vi "Acquire_PID_Tests.vi"() -> ()   [LabVIEW 2016]
panel:
  in  "Wait For Microscope?":bool
  in  "stop2":bool
  in  "Flow Path":path=path "E:/maggot images/Jacob/20171101/Flow_tests_run101.txt"
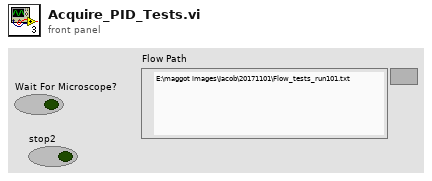
[diagram p1: front panel]
types:
  T1 = cluster{"relative seconds":dbl, "Pressures":dbl[], "F1 PID gains":dbl[], "FTot PID gains":dbl[], "PID On?":i16, "flow setpoints":dbl[]}
  T2 = cluster{"Time":dbl, "All Flow-Rates":dbl[], "Flow 2 Filter Time":dbl, "Flow 1 Filter Time":dbl}
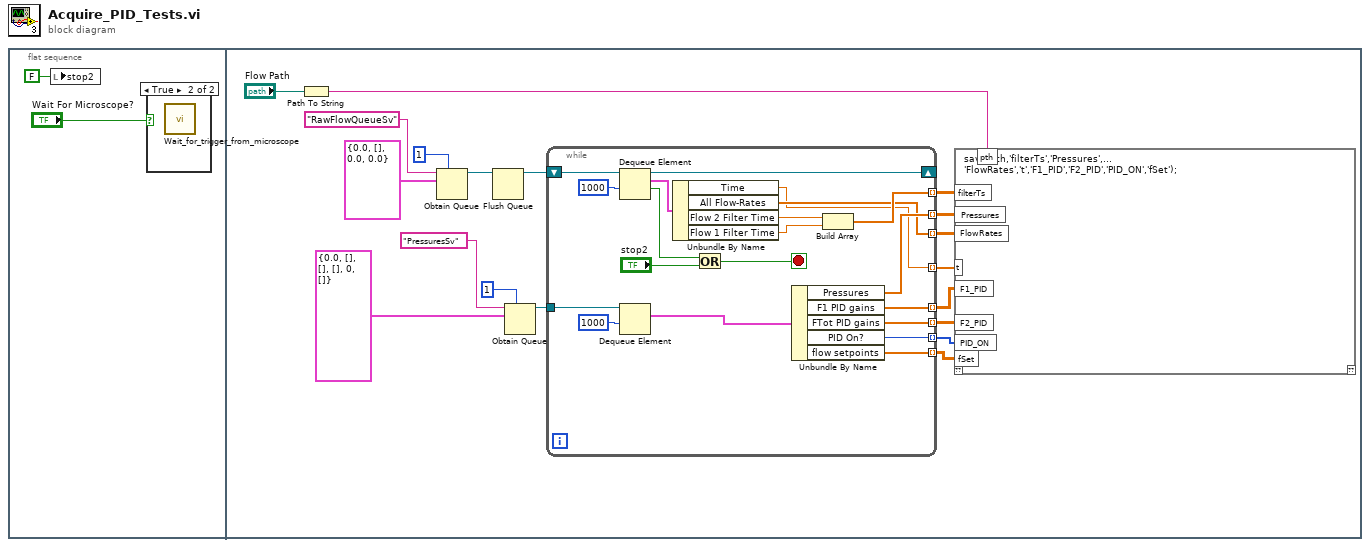
[diagram p0: block diagram]
diagram:
  n1 = flat-sequence {
    frame #0 {
      n2 = local write "stop2"(FALSE ("stop2")) -> ()
      n3 = case shown="True" "Wait For Microscope?" {
        frame False {
        }
        frame True {
          n4 = call "Wait_for_trigger_from_microscope.vi"() -> ()  [unwired: 12 in]
        }
      }
    }
    frame #1 {
      n5 = Path To String(path="Flow Path") -> (string=w5:string)
      n6 = Obtain Queue(max queue size (-1, unlimited)=1, name (unnamed)="RawFlowQueueSv", element data type=T2 {"Time"=0.0, "All Flow-Rates"=[], "Flow 2 Filter Time"=0.0, "Flow 1 Filter Time"=0.0} ("output cluster")) -> (queue out=w20:refnum<queue>)  [unwired: 2 in, 2 out]
      n7 = Flush Queue(queue=w20) -> (queue out=w19:refnum<queue>)  [unwired: 1 in, 2 out]
      n8 = Obtain Queue(max queue size (-1, unlimited)=1, name (unnamed)="PressuresSv", element data type=T1 {"relative seconds"=0.0, "Pressures"=[], "F1 PID gains"=[], "FTot PID gains"=[], "PID On?"=0, "flow setpoints"=[]} ("output cluster")) -> (queue out=w15:refnum<queue>)  [unwired: 2 in, 2 out]
      n9 = while {
        shift-right: [w38] -> _
        shift-left: w19 -> [w41]
        tunnel: w15 -> [w34]
        tunnel: [w29] -> w6 mode=indexing
        tunnel: [w28] -> w7 mode=indexing
        tunnel: [w27] -> w8 mode=indexing
        tunnel: [w26] -> w10 mode=indexing
        tunnel: [w25] -> w12 mode=indexing
        tunnel: [w24] -> w11 mode=indexing
        tunnel: [w23] -> w9 mode=indexing
        tunnel: [w22] -> w3 mode=indexing
        stop <- w37 stop-if-true
        n10 = Dequeue Element(queue=w41, timeout in ms (-1)=1000) -> (queue out=w38:refnum<queue>, element=w33:T2, timed out?=w39:bool)  [unwired: 1 in, 1 out]
        n11 = Dequeue Element(queue=w34, timeout in ms (-1)=1000) -> (element=w30:T1)  [unwired: 1 in, 3 out]
        n12 = Unbundle By Name(w33) -> ("Time"=w23:dbl, "All Flow-Rates"=w24:dbl[], "Flow 2 Filter Time"=w32:dbl, "Flow 1 Filter Time"=w31:dbl)
        n13 = Or(x=w39, y="stop2") -> (x .or. y?=w37:bool)
        n14 = Unbundle By Name(w30) -> ("Pressures"=w26:dbl[], "F1 PID gains"=w27:dbl[], "FTot PID gains"=w28:dbl[], "PID On?"=w29:i16, "flow setpoints"=w22:dbl[])
        n15 = Build Array(w32, w31) -> (w25:dbl[])
      }
      n16 = script code="save(pth,'filterTs','Pressures',...\n'FlowRates','t','F1_PID','F2_PID','PID_ON','fSet');"("pth"=w5, "t"=w9, "F1_PID"=w8, "F2_PID"=w7, "PID_ON"=w6, "Pressures"=w10, "FlowRates"=w11, "filterTs"=w12, "fSet"=w3) -> ()  [unwired: 1 in, 1 out]
    }
  }
